vi "Player Info.vi"(11 "BTeam in":refnum<class "BTeam.lvclass">) -> (1 "Victory Speach":string="There is no 'I' in TEAM!", 2 "Name":string="Team Effort!", 3 "BTeam out":refnum<class "BTeam.lvclass">)   [LabVIEW 2015, in "BTeam.lvclass"]
uses:
  BTeam.lvclass
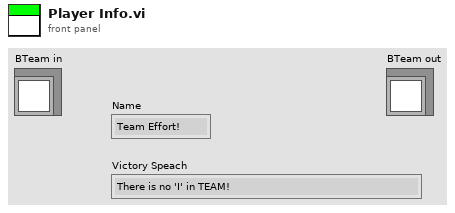
[diagram p1: front panel]
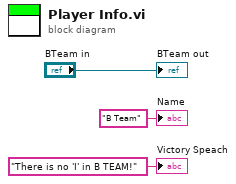
[diagram p0: block diagram]
diagram:
  "BTeam out" <- "BTeam in"
  "Name" <- "B Team" ("Name")
  "Victory Speach" <- "There is no 'I' in B TEAM!" ("Victory Speach")
